vi "End_Effector_State.vi"(4 "node":string, 5 "error in":errorcluster, 6 "Delay":u32, 8 "Side":T1) -> (0 "error out":errorcluster, 1 "force":sgl, 2 "position":sgl, 3 "Reply":string)   [LabVIEW 2013]
doc: "This will open or close the gripper to a specific position"
uses:
  ROS/Code/SubVIs/BaxterSide.ctl
  ROS/Code/_ROSDefinition.vi
panel:
  out "error out 2":errorcluster
  out "Reply 2":string
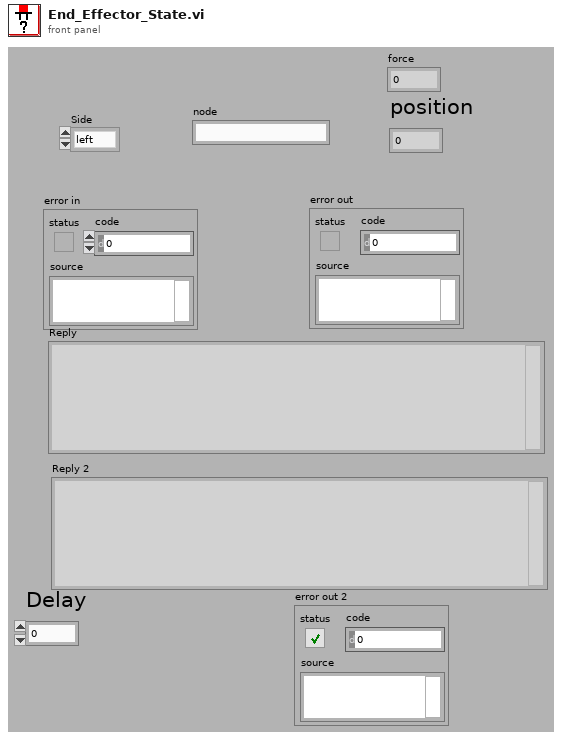
[diagram p1: front panel]
types:
  T1 = typedef "BaxterSide.ctl" = enum16{"left", "right"}
  T2 = enum16{"big-endian, network order", "native, host order", "little-endian"}
  T3 = typedef "_ROSControl.ctl" = cluster{"topic port":u16, "Node":string, "topic":string, "type":string, "node port":u32, "error ":errorcluster, "Direction":T4, "APIs":string[]}
  T4 = typedef "_ROSDirection.ctl" = enum16{"Node", "Publisher", "Subscriber", "Service Client"}
  T5 = cluster{"Seconds":u32, "NanoSec":u32, "ID":u32, "enabled":enum8{"FALSE", "TRUE", "UNKNOWN"}, "calibrated":enum8{"FALSE", "TRUE", "UNKNOWN"}, "ready":enum8{"FALSE", "TRUE", "UNKNOWN"}, "moving":enum8{"FALSE", "TRUE", "UNKNOWN"}, "gripping":enum8{"FALSE", "TRUE", "UNKNOWN"}, "missed":enum8{"FALSE", "TRUE", "UNKNOWN"}, "error":enum8{"FALSE", "TRUE", "UNKNOWN"}, "reverse":enum8{"FALSE", "TRUE", "UNKNOWN"}, "position":sgl, "force":sgl, "state":string, "command":string, "command sender":string, "command sequence":u32}
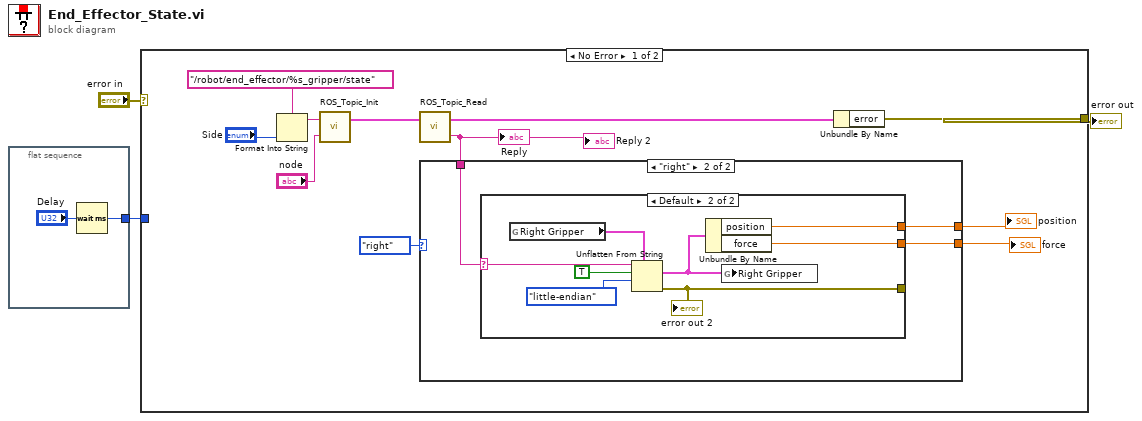
[diagram p0: block diagram]
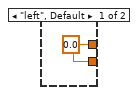
[diagram p2: hidden frame]
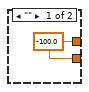
[diagram p3: hidden frame]
diagram:
  n1 = flat-sequence {
    tunnel: [w5] -> w1
    frame #0 {
      n2 = Wait (ms)(milliseconds to wait="Delay") -> (millisecond timer value=w5:u32)
    }
  }
  n3 = case shown="No Error" "error in" {
    selector: "error in" -> [_ w30]
    tunnel: [w16 w30] -> w3
    tunnel: w1 -> [_ _]
    frame No Error {
      n4 = Format Into String(format string="/robot/end_effector/%s_gripper/state" ("topic"), "Side") -> (resulting string=w14:string)  [unwired: 2 in, 1 out]
      n5 = call "ROS_Topic_Init.vi"("node"="node", "topic"=w14) -> ("ROS out"=w12:T3)  [unwired: 1 in]
      n6 = call "ROS_Topic_Read.vi"("ROS in"=w12) -> ("Reply"=w10:string, "ROS out"=w11:T3)  [unwired: 1 in]
      "Reply" <- w10
      "Reply 2" <- w10
      n7 = case shown="\"right\"" BaxterSide."right" ("Side") {
        tunnel: w10 -> [_ w20]
        tunnel: [w17 w19] -> w7
        tunnel: [w17 w18] -> w6
        frame "left", Default {
          w17 = sgl 0.0 ("position")
        }
        frame "right" {
          n8 = case shown="Default" w20 {
            selector: w20 -> [_ w29]
            tunnel: [_ w26] -> _
            tunnel: [w21 w23] -> w19
            tunnel: [w21 w22] -> w18
            frame "" {
              w21 = sgl -100.0 ("position")
            }
            frame Default {
              n9 = global read "_ROSDefinition.vi" "Right Gripper"() -> (w28:T5)
              n10 = Unflatten From String(type=w28, binary string=w29, data includes array or string size? (T)=TRUE, byte order (0:big-endian, network order)=T2."little-endian") -> (value=w24:T5, error out=w26:errorcluster)  [unwired: 1 in, 1 out]
              "error out 2" <- w26
              n11 = Unbundle By Name(w24) -> ("position"=w23:sgl, "force"=w22:sgl)
              n12 = global write "_ROSDefinition.vi" "Right Gripper"(w24) -> ()
            }
          }
        }
      }
      "position" <- w7
      "force" <- w6
      n13 = Unbundle By Name(w11) -> ("error"=w16:errorcluster)
    }
    frame Error {
    }
  }
  "error out" <- w3
